vi "Image Processing.vi"() -> ()   [LabVIEW 2012]
uses:
  <vilib>/picture/picture.llb/imagedata.ctl
panel:
  out "new picture":picture
  in  "path to JPEG file":path
  out "path 2":path
  out "Output Array":dbl[](array[numeric])
  out "Array 2":dbl[](array[numeric])
  out "Numeric 2":i32
  out "reversed array":i8[](array[numeric])
  out "output array 3":i8[][](array[numeric])
  out "output array 2":i8[](array[numeric])
  out "0, 2":i16[][](array[numeric])
  out "image 2":u8[](array[numeric])
  out "image":u8[](array[numeric])
  out "image data":T1
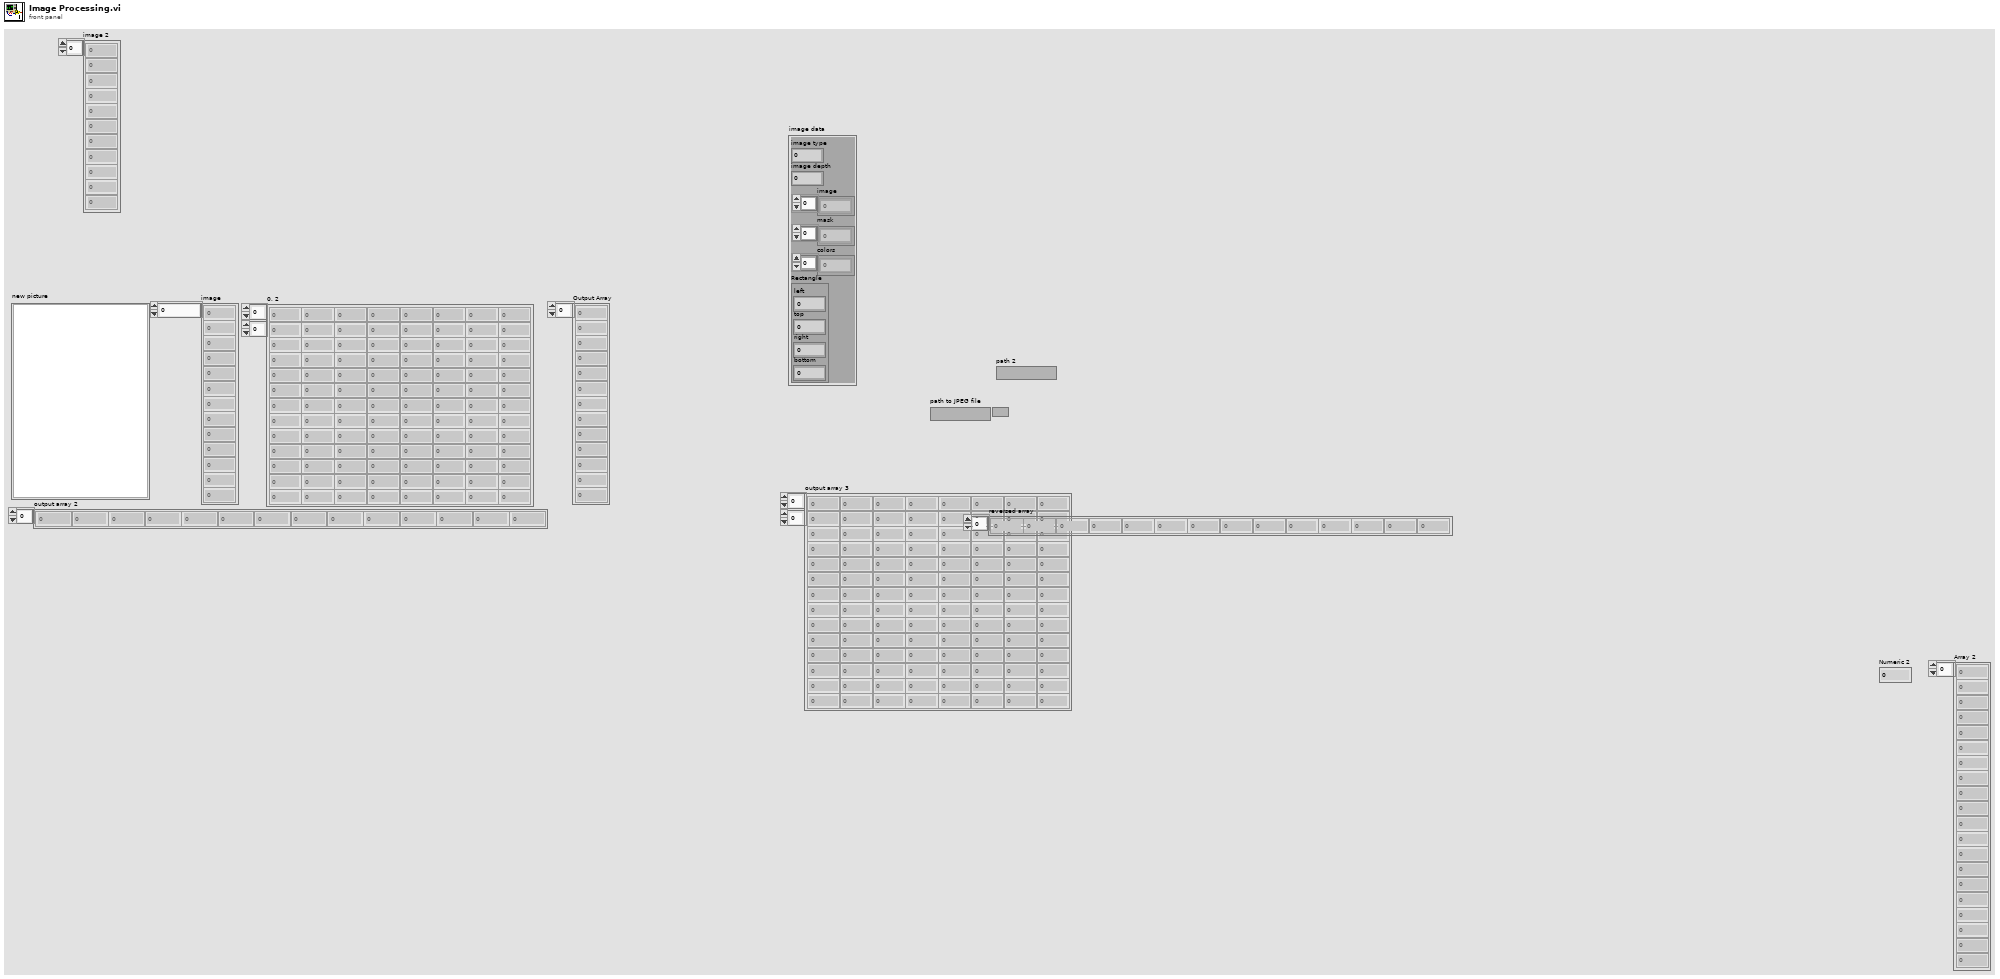
[diagram p1: front panel]
types:
  T1 = typedef "imagedata.ctl" = cluster{"image type":i32, "image depth":i32, "image":u8[], "mask":u8[], "colors":u32[], "Rectangle":cluster{"left":i16, "top":i16, "right":i16, "bottom":i16}}
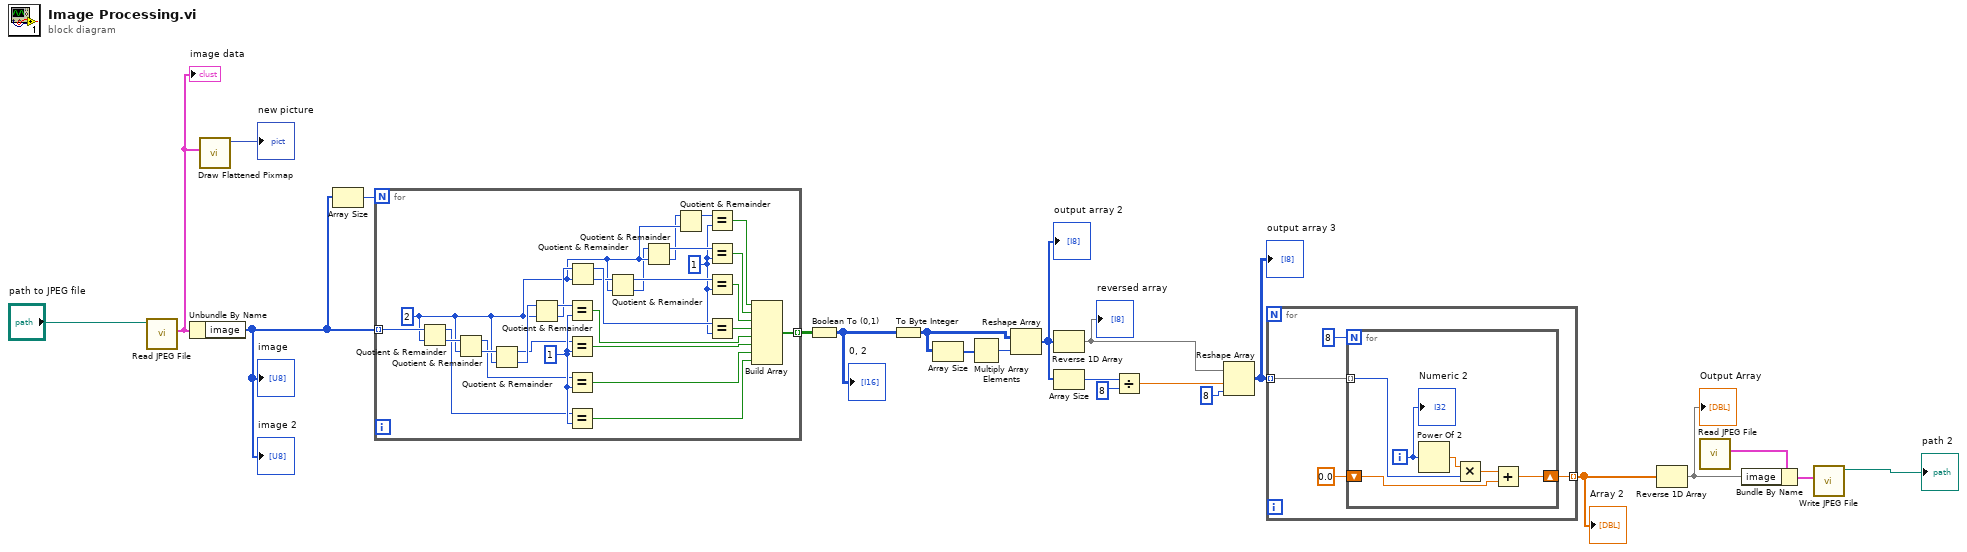
[diagram p0: block diagram]
diagram:
  n1 = call <vilib>:"Read JPEG File.vi"("path to JPEG file"="path to JPEG file") -> ("image data"=w4:T1)  [unwired: 8 in, 2 out]
  "image data" <- w4
  n2 = Unbundle By Name(w4) -> ("image"=w5:u8[])
  "image" <- w5
  "image 2" <- w5
  n3 = call <vilib>:"Draw Flattened Pixmap.vi"("image data"=w4) -> ("new picture"=→"new picture":picture)  [unwired: 8 in]
  n4 = Array Size(array=w5) -> (size(s)=w22:i32)
  n5 = for {
    N: w22 -> [_]
    tunnel: w5 -> [w46] mode=indexing
    tunnel: [w23] -> w21 mode=indexing
    w37 = 1
    w34 = 2
    w47 = 1
    n6 = Quotient & Remainder(x=w46, y=w34) -> (x-y*floor(x/y)=w45:i32, floor(x/y)=w48:i32)
    n7 = Quotient & Remainder(x=w48, y=w34) -> (x-y*floor(x/y)=w44:i32, floor(x/y)=w49:i32)
    n8 = Quotient & Remainder(x=w49, y=w34) -> (x-y*floor(x/y)=w43:i32, floor(x/y)=w50:i32)
    n9 = Quotient & Remainder(x=w50, y=w34) -> (x-y*floor(x/y)=w42:i32, floor(x/y)=w35:i32)
    n10 = Equal?(x=w42, y=w47) -> (x = y?=w27:bool)
    n11 = Equal?(x=w43, y=w47) -> (x = y?=w26:bool)
    n12 = Equal?(x=w44, y=w47) -> (x = y?=w25:bool)
    n13 = Equal?(x=w45, y=w47) -> (x = y?=w24:bool)
    n14 = Quotient & Remainder(x=w35, y=w34) -> (x-y*floor(x/y)=w38:i32, floor(x/y)=w36:i32)
    n15 = Quotient & Remainder(x=w36, y=w34) -> (x-y*floor(x/y)=w39:i32, floor(x/y)=w33:i32)
    n16 = Quotient & Remainder(x=w33, y=w34) -> (x-y*floor(x/y)=w40:i32, floor(x/y)=w32:i32)
    n17 = Quotient & Remainder(x=w32, y=w34) -> (x-y*floor(x/y)=w41:i32)  [unwired: 1 out]
    n18 = Equal?(x=w41, y=w37) -> (x = y?=w31:bool)
    n19 = Equal?(x=w40, y=w37) -> (x = y?=w30:bool)
    n20 = Equal?(x=w39, y=w37) -> (x = y?=w29:bool)
    n21 = Equal?(x=w38, y=w37) -> (x = y?=w28:bool)
    n22 = Build Array(w31, w30, w29, w28, w27, w26, w25, w24) -> (w23:bool[])
  }
  n23 = Boolean To (0,1)(Boolean=w21) -> (0, 1=w1:i16[][])
  "0, 2" <- w1
  n24 = To Byte Integer(number=w1) -> (8bit integer=w18:i8[][])
  n25 = Array Size(array=w18) -> (size(s)=w20:i32[])
  n26 = Multiply Array Elements(1:w20) -> (0:w19:i32)
  n27 = Reshape Array(w18, w19) -> (w13:i8[])
  "output array 2" <- w13
  n28 = Reverse 1D Array(array=w13) -> (reversed array=w12:i8[])
  "reversed array" <- w12
  n29 = Array Size(array=w13) -> (size(s)=w17:i32)
  n30 = Divide(x=w17, y=8) -> (x/y=w14:dbl)
  n31 = Reshape Array(w12, w14, 8 ("dimension size")) -> (w11:i8[][])
  "output array 3" <- w11
  n32 = for {
    tunnel: [w52] -> w10 mode=indexing
    tunnel: w11 -> [w51] mode=indexing
    n33 = for {
      N: 8 -> [_]
      shift-right: [w58] -> w52
      shift-left: 0.0 -> [w59]
      tunnel: w51 -> [w55] mode=indexing
      i -> [w57]
      n34 = Power Of 2(x=w57) -> (2^x=w56:dbl)
      n35 = Multiply(x=w56, y=w55) -> (x*y=w60:dbl)
      n36 = Add(x=w60, y=w59) -> (x+y=w58:dbl)
      "Numeric 2" <- w57
    }
  }
  "Array 2" <- w10
  n37 = Reverse 1D Array(array=w10) -> (reversed array=w8:dbl[])
  "Output Array" <- w8
  n38 = call <vilib>:"Read JPEG File.vi"() -> ("image data"=w9:T1)  [unwired: 9 in, 2 out]
  n39 = Bundle By Name(cluster=w9, "image"=w8) -> (w7:T1)
  n40 = call <vilib>:"Write JPEG File.vi"("image data"=w7) -> ("path"=→"path 2":path)  [unwired: 9 in, 1 out]
